vi "Create Community Link Page.vi"() -> ()   [LabVIEW 2020]
uses:
  CategoriesEnum.ctl
panel:
  out "File Markdown Text":string
  in  "Image Path":path
  in  "Learn Something":bool caption="Checkbox"
  in  "Handle the Details":bool caption="Checkbox"
  in  "Get Code":bool caption="Checkbox"
  in  "Find Answers":bool caption="Checkbox"
  in  "Engage with Peers":bool caption="Checkbox"
  in  "Connect with Others":bool caption="Checkbox"
  in  "Full Description":string
  in  "External URL":string
  in  "Date":timestamp format="%<%.0X %x>T"
  in  "Summary":string
  in  "Title":string
  # "Category(ies)"
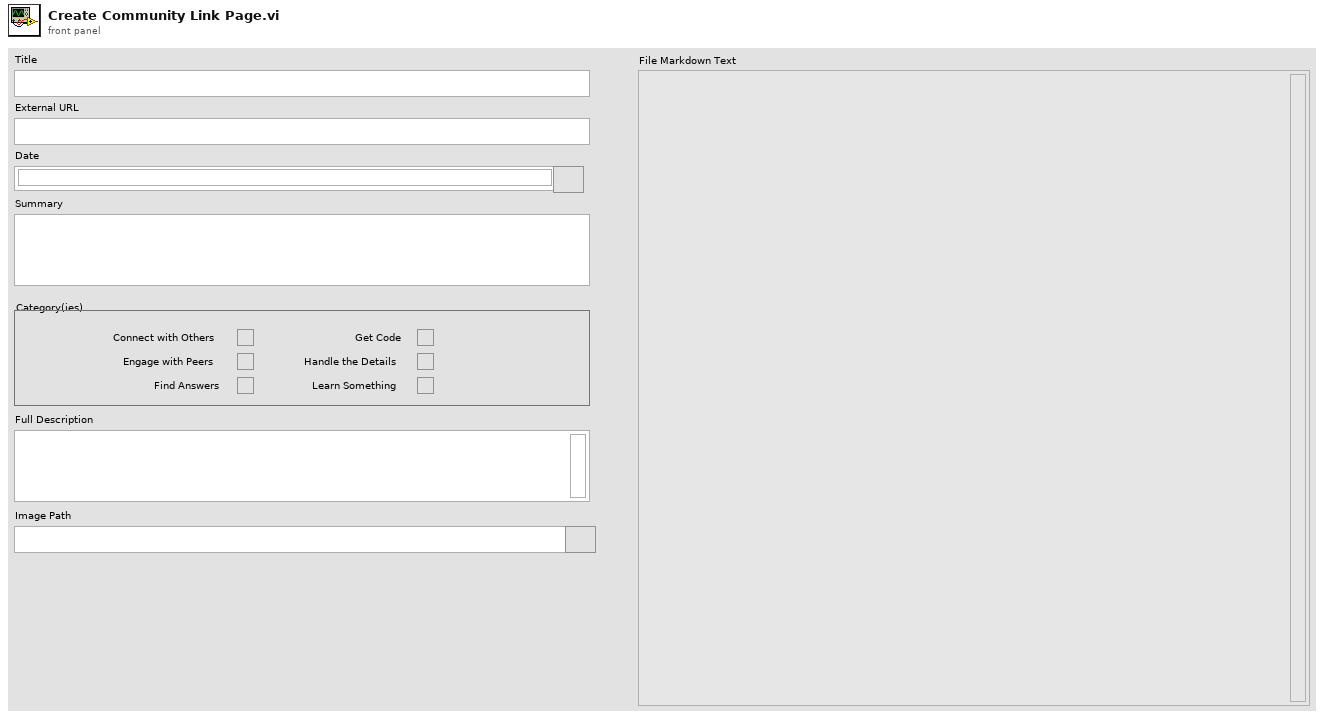
[diagram p1: front panel]
types:
  T1 = typedef "CategoriesEnum.ctl" = enum16{"Connect with Others", "Engage with Peers", "Find Answers", "Get Code", "Handle the Details", "Learn Something"}
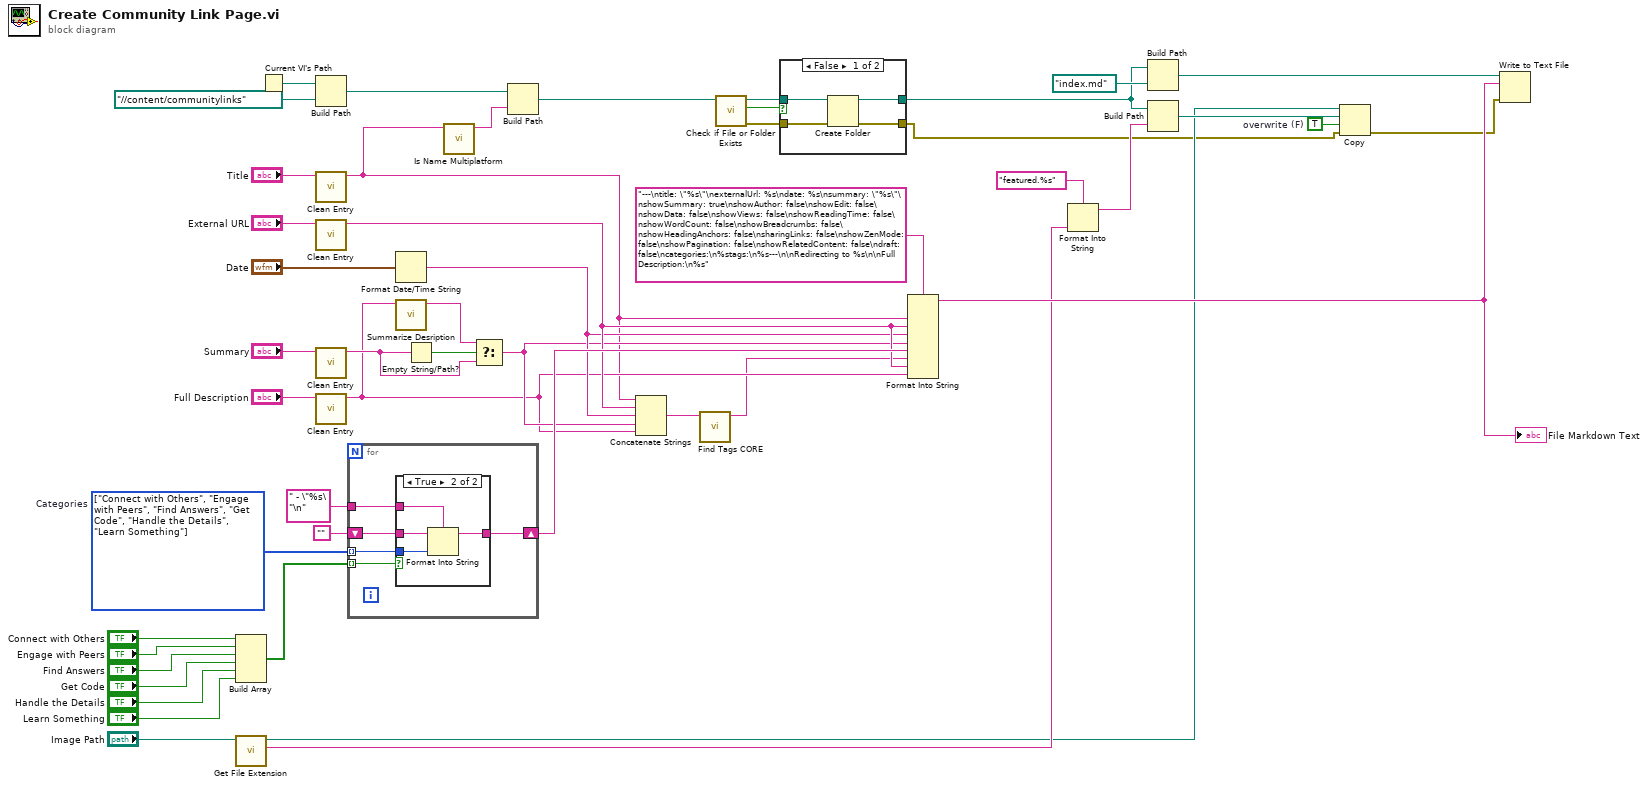
[diagram p0: block diagram]
diagram:
  w2 = TRUE  # overwrite (F)
  w24 = T1[] [enum."Connect with Others", enum."Engage with Peers", enum."Find Answers", enum."Get Code", enum."Handle the Details", enum."Learn Something"] items=["Connect with Others", "Engage with Peers", "Find Answers", "Get Code", "Handle the Details", "Learn Something"]  # Categories
  n1 = Build Array("Connect with Others", "Engage with Peers", "Find Answers", "Get Code", "Handle the Details", "Learn Something") -> (w23:bool[])
  n2 = call <vilib>:"Get File Extension.vi"("file"="Image Path") -> ("lowercase file extension"=w7:string, "dup file"=w6:path)  [unwired: 6 in, 3 out]
  n3 = Current VI's Path() -> (path=w48:path)
  n4 = Build Path(base path=w48, name or relative path=path "../../content/communitylinks") -> (appended path=w12:path)
  n5 = call "Clean Entry.vi"("string in"="Title") -> ("string out"=w1:string)  [unwired: 10 in]
  n6 = call "Clean Entry.vi"("string in"="External URL") -> ("string out"=w19:string)  [unwired: 10 in]
  n7 = call "Clean Entry.vi"("string in"="Summary") -> ("string out"=w31:string)  [unwired: 10 in]
  n8 = call "Clean Entry.vi"("string in"="Full Description") -> ("string out"=w16:string)  [unwired: 10 in]
  n9 = for {
    tunnel: w24 -> [w53] mode=indexing
    tunnel: w23 -> [w50] mode=indexing
    shift-right: [w52] -> w20
    shift-left: "" -> [w49]
    tunnel: " - \"%s\"\n" -> [w51]
    n10 = case shown="True" w50 {
      tunnel: w53 -> [_ w58]
      tunnel: [w54 w57] -> w52
      tunnel: w51 -> [_ w56]
      tunnel: w49 -> [w54 w55]
      frame False {
      }
      frame True {
        n11 = Format Into String(format string=w56, initial string=w55, w58) -> (resulting string=w57:string)  [unwired: 1 in, 1 out]
      }
    }
  }
  n12 = Format Date/Time String(seconds (now)="Date") -> (date/time string=w18:string)  [unwired: 2 in]
  n13 = call "Summarize Desription.vi"("Description in"=w16) -> ("Summary out"=w37:string)  [unwired: 10 in]
  n14 = Empty String/Path?(string/path=w31) -> (empty?=w38:bool)
  n15 = call <vilib>:"Is Name Multiplatform.vi"("filename"=w1) -> ("suggested filename"=w11:string)  [unwired: 6 in, 4 out]
  n16 = Select(t=w37, s=w38, f=w31) -> (s? t:f=w17:string)
  n17 = Build Path(base path=w12, name or relative path=w11) -> (appended path=w10:path)
  n18 = Concatenate Strings(w1, w19, w18, w17, w16) -> (w15:string)
  n19 = call "Find Tags CORE.vi"("Index"=w15) -> ("Tags Front Matter"=w14:string)  [unwired: 10 in]
  n20 = call <vilib>:"Check if File or Folder Exists.vi"("path"=w10) -> ("error out"=w46:errorcluster, "file or folder exists?"=w44:bool, "dup path"=w43:path)  [unwired: 8 in]
  n21 = case shown="False" w44 {
    tunnel: w43 -> [w60 w63]
    tunnel: [w59 w63] -> w40
    tunnel: w46 -> [w62 w64]
    tunnel: [w61 w64] -> w4
    frame False {
      n22 = Create Folder(path (use dialog)=w60, error in=w62) -> (created path=w59:path, error out=w61:errorcluster)  [unwired: 1 in, 1 out]
    }
    frame True {
    }
  }
  n23 = Format Into String(format string="---\ntitle: \"%s\"\nexternalUrl: %s\ndate: %s\nsummary: \"%s\"\nshowSummary: true\nshowAuthor: false\nshowEdit: false\nshowData: false\nshowViews: false\nshowReadingTime: false\nshowWordCount: false\nshowBreadcrumbs: false\nshowHeadingAnchors: false\nsharingLinks: false\nshowZenMode: false\nshowPagination: false\nshowRelatedContent: false\ndraft: false\ncategories:\n%stags:\n%s---\n\nRedirecting to %s\n\nFull Description:\n%s", w1, w19, w18, w17, w20, w14, w19, w16) -> (resulting string=w13:string)  [unwired: 2 in, 1 out]
  "File Markdown Text" <- w13
  n24 = Format Into String(format string="featured.%s", w7) -> (resulting string=w5:string)  [unwired: 2 in, 1 out]
  n25 = Build Path(base path=w40, name or relative path=path "index.md") -> (appended path=w41:path)
  n26 = Build Path(base path=w40, name or relative path=w5) -> (appended path=w39:path)
  n27 = Copy(8:w4, 9:w2, 10:w39, 11:w6) -> (0:w3:errorcluster)  [unwired: 1 in, 2 out]
  n28 = Write to Text File(file (use dialog)=w41, text=w13, error in=w3) -> ()  [unwired: 1 in, 3 out]
